vi "GZip_String_via_dotNet.vi"(3 "error in (no error)":errorcluster, 4 "Action":enum16{"Pack", "Unpack"}(ring), 5 "String Input":string) -> (0 "error out":errorcluster, 1 "(Un)pack ratio":dbl, 2 "String Output (GZipped/UnGZipped)":string)   [LabVIEW 2018, in "Tracker.lvlib"]
uses:
  Tracker.lvlib
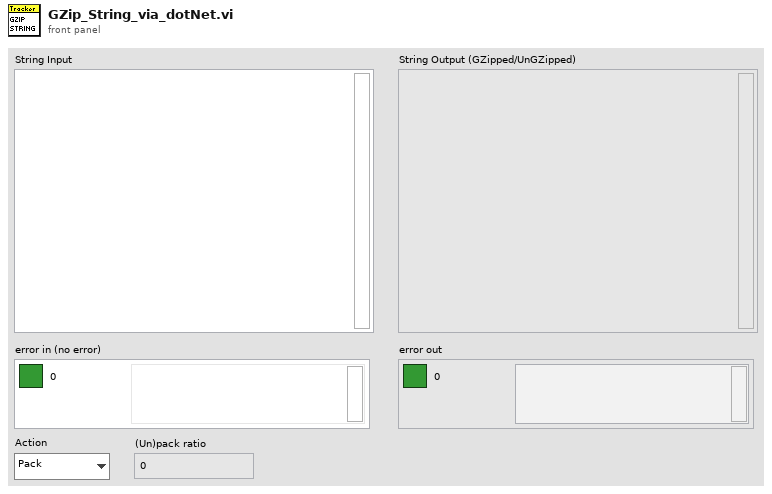
[diagram p1: front panel]
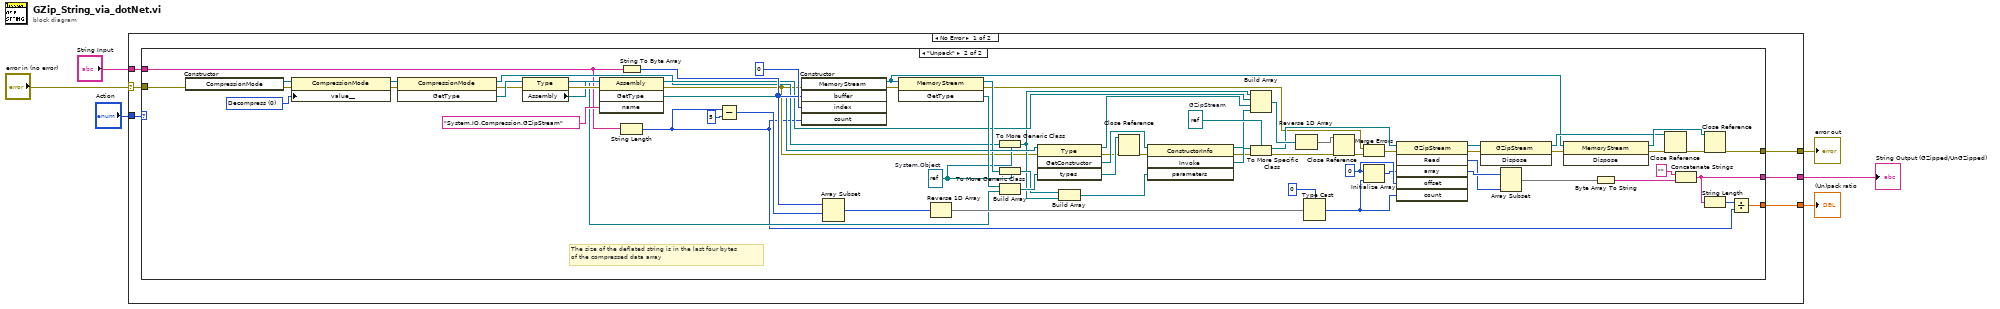
[diagram p0: block diagram]
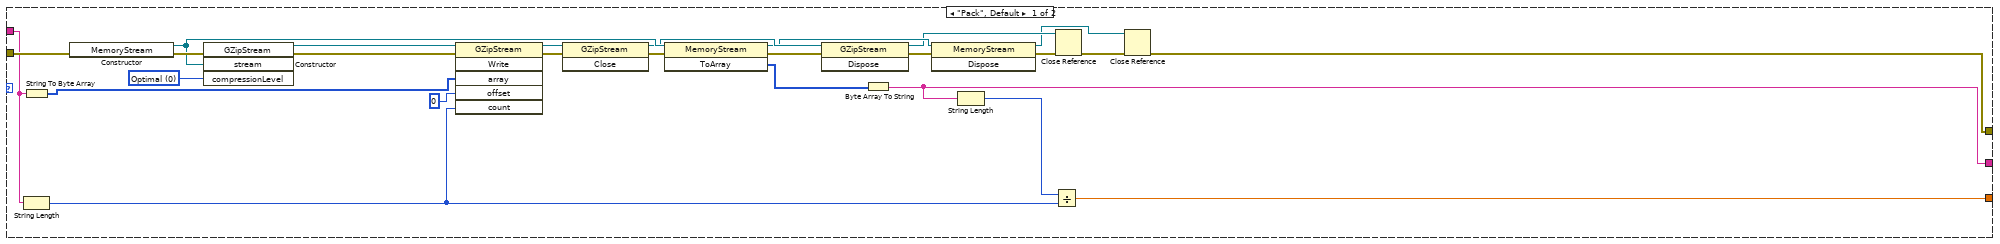
[diagram p2: hidden frame]
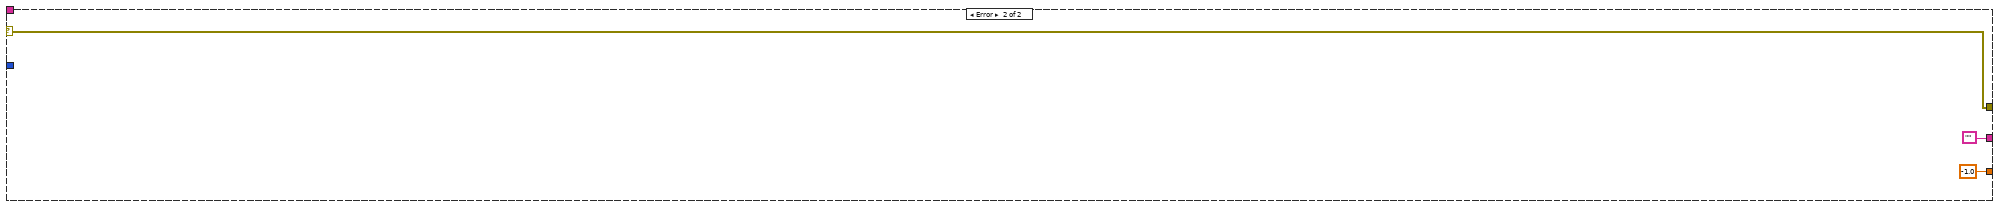
[diagram p3: hidden frame]
diagram:
  n1 = case shown="No Error" "error in (no error)" {
    selector: "error in (no error)" -> [w12 w110]
    tunnel: [w7 w110] -> w5
    tunnel: "String Input" -> [w10 _]
    tunnel: [w9 ""] -> w3
    tunnel: [w8 -1.0] -> w2
    tunnel: "Action" -> [w11 _]
    frame No Error {
      n2 = case shown="\"Unpack\"" w11 {
        tunnel: w12 -> [w38 w44]
        tunnel: w10 -> [w31 w45]
        tunnel: [w15 w42] -> w9
        tunnel: [w14 w39] -> w8
        tunnel: [w13 w43] -> w7
        frame "Pack", Default {
          w36 = 0 items=["Optimal", "Fastest", "NoCompression"] ("compressionLevel")
          n3 = String To Byte Array(string=w31) -> (unsigned byte array=w33:u8[])
          n4 = String Length(string=w31) -> (length=w17:i32)
          n5 = constructor class="MemoryStream"(error in=w38) -> (reference out=w28:refnum<k24>, error out=w37:errorcluster)  [unwired: 2 in, 1 out]
          n6 = constructor class="GZipStream"(error in=w37, "stream"=w28, "compressionLevel"=w36) -> (reference out=w35:refnum<k24>, error out=w34:errorcluster)  [unwired: 2 in, 3 out]
          n7 = invoke class="GZipStream" method="Write"(reference=w35, error in=w34, "array"=w33, "offset"=0, "count"=w17) -> (reference out=w29:refnum<k24>, error out=w30:errorcluster)  [unwired: 1 in, 4 out]
          n8 = invoke class="GZipStream" method="Close"(reference=w29, error in=w30) -> (reference out=w25:refnum<k24>, error out=w27:errorcluster)  [unwired: 1 in, 1 out]
          n9 = invoke class="MemoryStream" method="ToArray"(reference=w28, error in=w27) -> (reference out=w24:refnum<k24>, error out=w26:errorcluster, "ToArray"=w18:u8[])  [unwired: 1 in]
          n10 = invoke class="GZipStream" method="Dispose"(reference=w25, error in=w26) -> (reference out=w22:refnum<k24>, error out=w23:errorcluster)  [unwired: 1 in, 1 out]
          n11 = Byte Array To String(unsigned byte array=w18) -> (string=w15:string)
          n12 = invoke class="MemoryStream" method="Dispose"(reference=w24, error in=w23) -> (reference out=w19:refnum<k24>, error out=w21:errorcluster)  [unwired: 1 in, 1 out]
          n13 = String Length(string=w15) -> (length=w16:i32)
          n14 = Divide(x=w16, y=w17) -> (x/y=w14:dbl)
          n15 = Close Reference(reference=w22, error in (no error)=w21) -> (error out=w20:errorcluster)
          n16 = Close Reference(reference=w19, error in (no error)=w20) -> (error out=w13:errorcluster)
        }
        frame "Unpack" {
          w54 = 0 items=["Decompress", "Compress"] ("CompressionMode in")
          w47 = refnum<k24> refnum  # System.Object
          w69 = refnum<k24> refnum  # GZipStream
          w95 = u8 0 ("offset")
          # "The size of the deflated string is in the last four bytes \nof the compressed data array"
          n17 = constructor class="CompressionMode"(error in=w44) -> (reference out=w73:refnum<k24>, error out=w80:errorcluster)  [unwired: 2 in, 1 out]
          n18 = property class="CompressionMode"(reference=w73, error in=w80, "value__"=w54) -> (reference out=w72:refnum<k24>, error out=w74:errorcluster)
          n19 = invoke class="CompressionMode" method="GetType"(reference=w72, error in=w74) -> (reference out=w56:refnum<k24>, error out=w78:errorcluster, "GetType"=w79:refnum<k24>)  [unwired: 1 in]
          n20 = property class="Type"(reference=w79, error in=w78) -> (reference out=w75:refnum<k24>, error out=w77:errorcluster, "Assembly"=w76:refnum<k24>)
          n21 = invoke class="Assembly" method="GetType"(reference=w76, error in=w77, "name"="System.IO.Compression.GZipStream") -> (reference out=w57:refnum<k24>, error out=w46:errorcluster, "GetType"=w82:refnum<k24>)  [unwired: 1 in, 1 out]
          n22 = String To Byte Array(string=w45) -> (unsigned byte array=w86:u8[])
          n23 = String Length(string=w45) -> (length=w40:i32)
          n24 = Subtract(x=w40, y=5) -> (x-y=w103:i32)
          n25 = constructor class="MemoryStream"(error in=w46, "buffer"=w86, "index"=0, "count"=w40) -> (reference out=w53:refnum<k24>, error out=w52:errorcluster)  [unwired: 2 in, 4 out]
          n26 = Array Subset(array=w86, index=w103) -> (w104:u8[])  [unwired: 1 in]
          n27 = invoke class="MemoryStream" method="GetType"(reference=w53, error in=w52) -> (reference out=w62:refnum<k24>, error out=w48:errorcluster, "GetType"=w84:refnum<k24>)  [unwired: 1 in]
          n28 = Reverse 1D Array(array=w104) -> (reversed array=w105:u8[])
          n29 = To More Generic Class(target class=w47, reference=w56) -> (generic class reference=w55:refnum<k24>)
          n30 = To More Generic Class(target class=w47, reference=w62) -> (generic class reference=w61:refnum<k24>)
          n31 = Build Array(w84, w75) -> (w83:refnum<k24>[])
          n32 = invoke class="Type" method="GetConstructor"(reference=w82, error in=w46, "types"=w83) -> (reference out=w58:refnum<k24>, error out=w65:errorcluster, "GetConstructor"=w81:refnum<k24>, "types"=w66:refnum<k24>[])  [unwired: 1 in]
          n33 = Build Array(w61, w55) -> (w71:refnum<k24>[])
          n34 = Close Reference(reference=w66, error in (no error)=w65) -> (error out=w64:errorcluster)
          n35 = invoke class="ConstructorInfo" method="Invoke"(reference=w81, error in=w64, "parameters"=w71) -> (reference out=w59:refnum<k24>, error out=w68:errorcluster, "Invoke"=w70:refnum<k24>)  [unwired: 1 in, 1 out]
          n36 = Build Array(w55, w57, w58, w59) -> (w67:refnum<k24>[])
          n37 = To More Specific Class(target class=w69, reference=w70, error in=w68) -> (specific class reference=w51:refnum<k24>, error out=w63:errorcluster)
          n38 = Reverse 1D Array(array=w67) -> (reversed array=w60:refnum<k24>[])
          n39 = Type Cast(type=u32 0, x=w105) -> (*(type *) &x=w107:u32)
          n40 = Close Reference(reference=w60, error in (no error)=w63) -> (error out=w50:errorcluster)
          n41 = Merge Errors(w48, w50) -> (w49:errorcluster)
          n42 = Initialize Array(w95, w107) -> (w94:u8[])
          n43 = invoke class="GZipStream" method="Read"(reference=w51, error in=w49, "array"=w94, "offset"=w95, "count"=w107) -> (reference out=w97:refnum<k24>, error out=w98:errorcluster, "Read"=w91:i32, "array"=w96:u8[])  [unwired: 1 in, 2 out]
          n44 = invoke class="GZipStream" method="Dispose"(reference=w97, error in=w98) -> (reference out=w87:refnum<k24>, error out=w99:errorcluster)  [unwired: 1 in, 1 out]
          n45 = Array Subset(array=w96, length=w91) -> (w92:u8[])  [unwired: 1 in]
          n46 = invoke class="MemoryStream" method="Dispose"(reference=w53, error in=w99) -> (reference out=w90:refnum<k24>, error out=w89:errorcluster)  [unwired: 1 in, 1 out]
          n47 = Byte Array To String(unsigned byte array=w92) -> (string=w93:string)
          n48 = Close Reference(reference=w87, error in (no error)=w89) -> (error out=w88:errorcluster)
          n49 = Concatenate Strings("", w93) -> (w42:string)
          n50 = Close Reference(reference=w90, error in (no error)=w88) -> (error out=w43:errorcluster)
          n51 = String Length(string=w42) -> (length=w41:i32)
          n52 = Divide(x=w41, y=w40) -> (x/y=w39:dbl)
        }
      }
    }
    frame Error {
    }
  }
  "error out" <- w5
  "String Output (GZipped/UnGZipped)" <- w3
  "(Un)pack ratio" <- w2
